vi "Encode.vi"(8 "error in (no error)":errorcluster, 10 "String":string, 11 "Serializer.Base64 in":refnum<class "Serializer.Base64.lvclass">) -> (0 "error out":errorcluster, 2 "encoded string":string, 3 "Serializer.Base64 out":refnum<class "Serializer.Base64.lvclass">)   [LabVIEW 2013, in "Serializer.Base64.lvclass"]
doc: "Base64 encodes the string using the configured charset."
uses:
  Serializer.Base64.lvclass
  Serializer.Base64.lvclass/Serializer.Base64.ctl
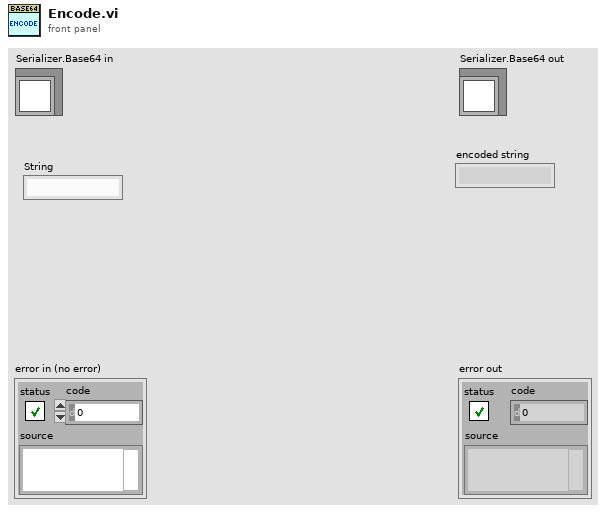
[diagram p1: front panel]
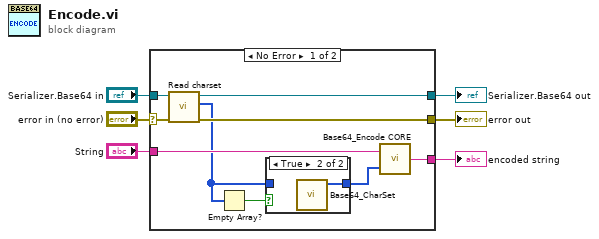
[diagram p0: block diagram]
diagram:
  n1 = case shown="No Error" "error in (no error)" {
    selector: "error in (no error)" -> [w13 w19]
    tunnel: [w12 w19] -> w5
    tunnel: [w11 w18] -> w3
    tunnel: "Serializer.Base64 in" -> [w10 w18]
    tunnel: "String" -> [w15 _]
    tunnel: [w14 _] -> w1
    frame No Error {
      n2 = call "Read charset.vi"("error in (no error)"=w13, "Serializer.Base64 in"=w10) -> ("error out"=w12:errorcluster, "charset"=w8:u8[], "Serializer.Base64 out"=w11:refnum<class "Serializer.Base64.lvclass">)  [unwired: 7 in]
      n3 = Empty Array?(array=w8) -> (empty?=w9:bool)
      n4 = case shown="True" w9 {
        tunnel: [w16 w17] -> w7
        tunnel: w8 -> [w16 _]
        frame False {
        }
        frame True {
          n5 = call "Base64_CharSet.vi"() -> ("base64 set"=w17:u8[])  [unwired: 11 in]
        }
      }
      n6 = call "Base64_Encode CORE.vi"("base64 set"=w7, "String"=w15) -> ("string"=w14:string)
    }
    frame Error {
    }
  }
  "error out" <- w5
  "Serializer.Base64 out" <- w3
  "encoded string" <- w1
